vi "Tester_Sample_Usage.vi"() -> ()   [LabVIEW 2021]
panel:
  out "Returned Tester Configuration":string[][](array[string])
  in  "Catalog Number\nto search":string
  in  "Path to Tester CSV File":path
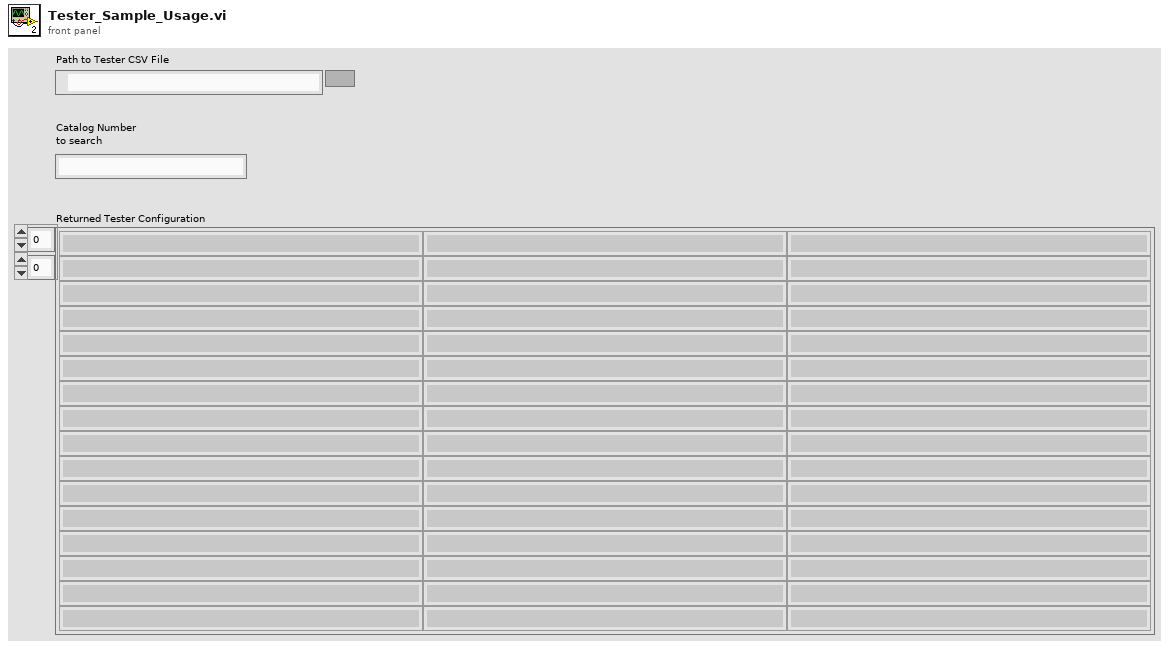
[diagram p1: front panel]
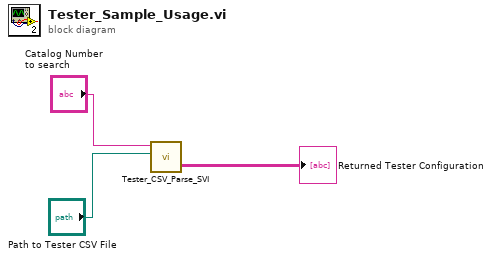
[diagram p0: block diagram]
diagram:
  n1 = call "Tester_CSV_Parse_SVI.vi"("Path to Tester CSV File"="Path to Tester CSV File", "Catalog Number\nto search"="Catalog Number\nto search") -> ("Final 2D \nOutput Array"=→"Returned Tester Configuration":string[][])  [unwired: 4 in, 5 out]
